vi "Waveform Gen.vi"(8 "reset":bool, 9 "samplesIn":i32=-1, 10 "RefIn":u32) -> (0 "timeString":string, 1 "dt":dbl, 2 "Y":dbl[](array[numeric]), 3 "error out":errorcluster, 4 "dateString":string, 5 "samplesOut":i32, 6 "waveform_state":i32, 7 "refOut":u32)   [LabVIEW 2021]
uses:
  <vilib>/addons/_NISVFA/_Generation/Signal Generation/SV Sinusoid/SV Sinusoid.lvclass
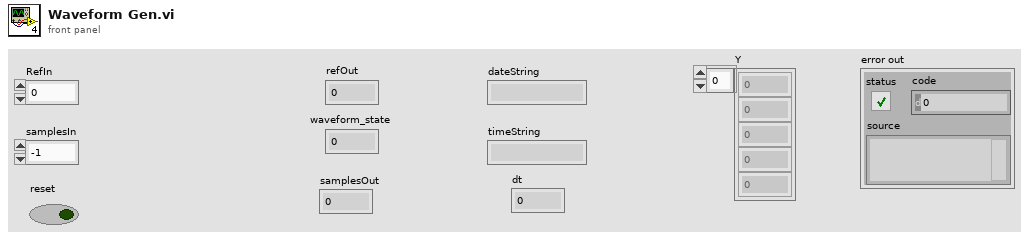
[diagram p1: front panel]
types:
  T1 = typedef "SV Signal.lvclass/sv_Generation State.ctl" = enum16{"Idle", "Ramp Up", "Pre-Measurement Settling", "Measurement", "Post-Measurement Settling", "Discrete Sweep Transition", "Ramp Down", "Update", "Leading Sync Pulse", "Trailing Sync Pulse"}
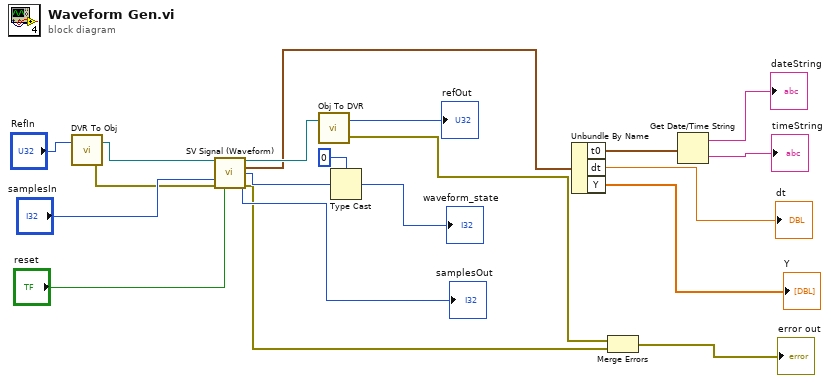
[diagram p0: block diagram]
diagram:
  n1 = call "DVR To Obj.vi"("RefIn"="RefIn") -> ("error_out"=w16:errorcluster, "data"=w20:refnum<class "SV Sinusoid.lvclass">)  [unwired: 1 in]
  n2 = call-dynamic "SV Signal (Waveform).vi"("signal configuration"=w20, "reset"="reset", "samples"="samplesIn", "error in (no error)"=w16) -> ("signal configuration"=w15:refnum<class "SV Sinusoid.lvclass">, "output waveform"=w9:waveform(dbl), "output waveform state"=w13:T1, "samples"=→"samplesOut":i32, "error out"=w2:errorcluster)  [unwired: 6 in, 1 out]
  n3 = call "Obj To DVR.vi"("signal configuration"=w15) -> ("error_out"=w3:errorcluster, "dataValueReference"=→"refOut":u32)  [unwired: 1 in]
  n4 = Type Cast(type=0 ("Numeric"), x=w13) -> (*(type *) &x=→"waveform_state":i32)
  n5 = Unbundle By Name(w9) -> ("t0"=w8:timestamp, "dt"=→"dt":dbl, "Y"=→"Y":dbl[])
  n6 = Merge Errors(w3, w2) -> (→"error out":errorcluster)
  n7 = Get Date/Time String(seconds (now)=w8) -> (date string=→"dateString":string, time string=→"timeString":string)  [unwired: 2 in]
